vi "Read any file Waveform 1ch.vi"(6 "Data type":waveform(dbl), 7 "tdms file in":refnum<k34>, 8 "error in":errorcluster, 9 "Data File Type":T2(ring), 10 "Data window":T1={"Start"=0, "Length"=500000, "Channel numbers"=[0], "Channel name"="", "Group name"="Untitled"}, 11 "Input file path":path) -> (0 "error out":errorcluster, 1 "1st channel length":u64, 2 "Data out":waveform(dbl), 3 "Actual input file path":path, 5 "tdms file out":refnum<k34>)   [LabVIEW 2021]
uses:
  ark_all/arkady-arxiv/oldTDOanalysis/Data window.ctl
panel:
  # "OR"
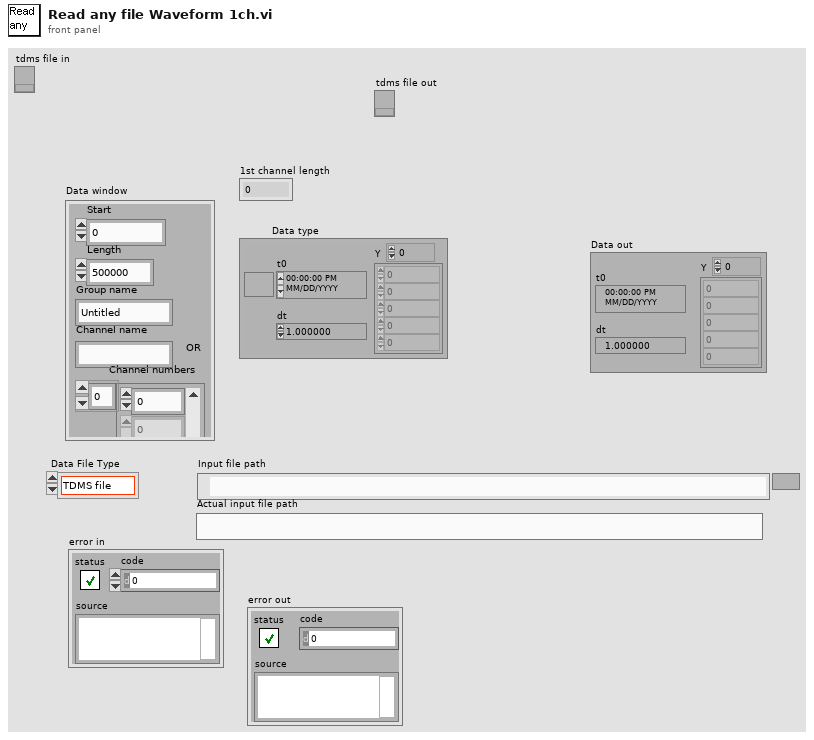
[diagram p1: front panel]
types:
  T1 = typedef "Data window.ctl" = cluster{"Start":i64, "Length":i64, "Channel numbers":i64[], "Channel name":string, "Group name":string}
  T2 = enum16{"TDMS file", "Tektronics ISF", "BinF file", "ASCII File", "BinH File", "BinW File", "BINARY File"}
  T3 = enum16{"open", "open or create", "create or replace", "create", "open (read-only)"}
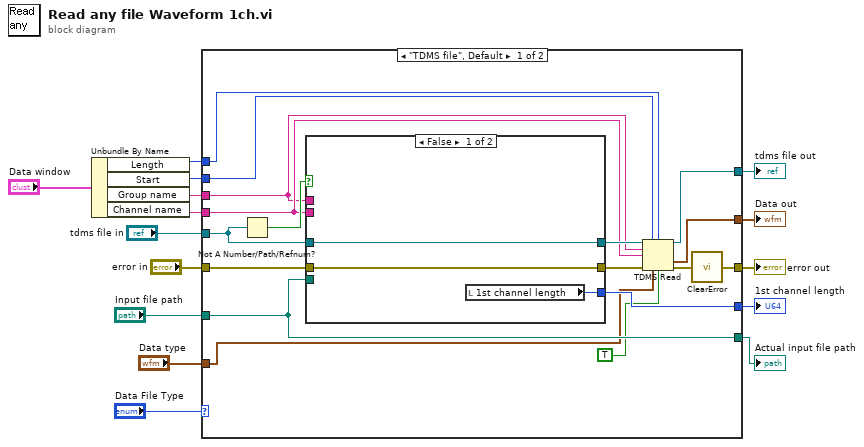
[diagram p0: block diagram]
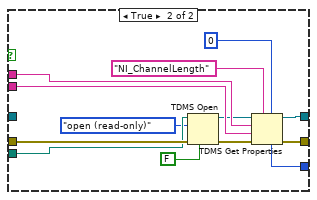
[diagram p2: hidden frame]
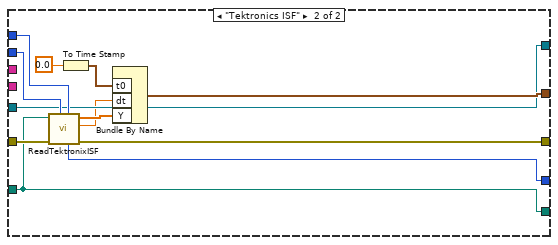
[diagram p3: hidden frame]
diagram:
  n1 = Unbundle By Name("Data window") -> ("Length"=w11:i64, "Start"=w1:i64, "Group name"=w8:string, "Channel name"=w10:string)
  n2 = case shown="\"TDMS file\", Default" "Data File Type" {
    tunnel: "Input file path" -> [w27 w53]
    tunnel: [w27 w53] -> w13
    tunnel: "error in" -> [w32 w56]
    tunnel: [w22 w55] -> w6
    tunnel: w1 -> [w29 w57]
    tunnel: w11 -> [w28 w58]
    tunnel: [w23 w51] -> w3
    tunnel: w10 -> [w20 _]
    tunnel: [w21 w52] -> w9
    tunnel: w8 -> [w19 _]
    tunnel: [w26 w50] -> w5
    tunnel: "tdms file in" -> [w24 w50]
    tunnel: "Data type" -> [w17 _]
    frame "TDMS file", Default {
      n3 = Not A Number/Path/Refnum?(number/path/refnum=w24) -> (NaN/Path/Refnum?=w25:bool)
      n4 = case shown="False" w25 {
        tunnel: w32 -> [w34 w48]
        tunnel: [w35 w37] -> w31
        tunnel: [w34 w42] -> w30
        tunnel: w27 -> [_ w47]
        tunnel: w24 -> [w35 _]
        tunnel: [w33 w41] -> w21
        tunnel: w20 -> [_ w40]
        tunnel: w19 -> [_ w39]
        frame False {
          n5 = local read "1st channel length"() -> (w33:u64)
        }
        frame True {
          n6 = TDMS Open(6:FALSE ("disable buffering (T)"), 8:w48, 10:T3."open (read-only)" ("operation (0:open)"), 11:w47) -> (0:w43:errorcluster, 3:w38:refnum<k34>)  [unwired: 3 in]
          n7 = TDMS Get Properties(5:u64 0, 7:"NI_ChannelLength" ("property name"), 8:w43, 9:w40, 10:w39, 11:w38) -> (0:w42:errorcluster, 3:w37:refnum<k34>, 4:w41:u64)  [unwired: 3 out]
        }
      }
      n8 = TDMS Read(0:w31, 1:w29, 2:w28, 5:w19, 7:w20, 11:w30, 12:w17, 13:TRUE ("return channels in file order? (F)")) -> (4:w26:refnum<k34>, 10:w23:waveform(dbl), 15:w18:errorcluster)  [unwired: 3 out]
      n9 = call <vilib>:"ClearError.vi"("error in (no error)"=w18) -> ("error out"=w22:errorcluster)
    }
    frame "Tektronics ISF" {
      n10 = call "ReadTektronixISF.vi"("Length"=w58, "Start"=w57, "error in (no error)"=w56, "Path"=w53) -> ("error out"=w55:errorcluster, "dt"=w49:dbl, "Data"=w54:dbl[], "Total number of points"=w52:u64)  [unwired: 4 out]
      n11 = To Time Stamp(1:0.0) -> (0:w59:timestamp)
      n12 = Bundle By Name("t0"=w59, "dt"=w49, "Y"=w54) -> (w51:waveform(dbl))  [unwired: 1 out]
    }
  }
  "Actual input file path" <- w13
  "error out" <- w6
  "1st channel length" <- w9
  "tdms file out" <- w5
  "Data out" <- w3
